vi "Signals.Scale.EU.vi"(4 "Buffer?":bool, 5 "Lookup":variant, 6 "Type":T1, 7 "Reads Ref":T2, 8 "error in (no error)":errorcluster, 10 "Unscaled Data":u8[](array[numeric]), 11 "ID":u32) -> (0 "error out":errorcluster)   [LabVIEW 2019, in "Diagnostics Addon Engine.lvlib"]
uses:
  Diagnostics Addon Engine.lvlib
  <vilib>/NI/NIVS Inline Async API/_Data Access Engine/Data Access Engine/Types/Write.DVR.ctl
  <vilib>/NI/NIVS Inline Async API/_Data Access Engine/Access Type Classes/Write/Write.lvclass
  Shared/Types/Type.ctl
  <vilib>/xnet/xnet.llb/XNET Frame CAN.ctl
  <vilib>/xnet/xnet.llb/XNET Frame Type CAN.ctl
  Shared/Types/Frame.Lookup.Info.ctl
  <vilib>/NI/NIVS Inline Async API/_Data Access Engine/Access Type Classes/Write/Write.lvclass/Write.ctl
  <vilib>/NI/NIVS Inline Async API/_Data Access Engine/Data Access Engine/Methods/Write.Data.Buffer.vi
  <vilib>/NI/NIVS Inline Async API/_Data Access Engine/Data Access Engine/Methods/Write.Data.vi
  <vilib>/NI/NIVS Inline Async API/_Data Access Engine/Access Type Classes/Write/Write.Buffer.vi
  <vilib>/NI/NIVS Inline Async API/_Data Access Engine/Access Type Classes/Write/Write.ProcessData.vi
  Shared/SubVIs/Constants.vi
  <vilib>/xnet/xnet.llb/XNET Convert (Frame CAN to Signal).vi
  Shared/Diagnostics Addon Shared.lvlib
  <vilib>/NI VeriStand/Custom Device Tools/Custom Device Utility Library/Custom Device Utility Library.lvlib
  <vilib>/NI/NIVS Inline Async API/_Data Access Engine/Data Access Engine/Data Access Engine.lvclass
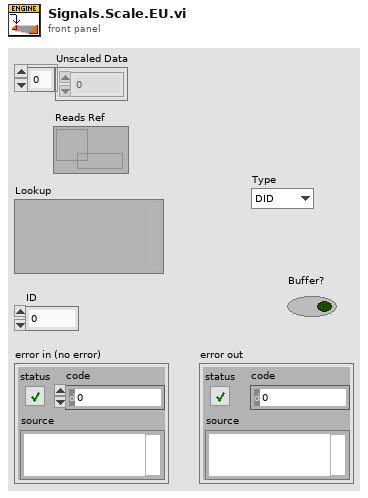
[diagram p1: front panel]
types:
  T1 = typedef "Diagnostics Addon Shared.lvlib/Type.ctl" = enum16{"DID", "CDID", "PID", "CPID", "Read Memory", "Write Memory", "IO Control", "Routine Start", "Routine Request", "Routine Stop", "User Defined", "DTC Control", "Clear DTCs", "Read DTCs", "Start DTCs", "DTC Change Count", "Tester Present", "Unlock ECU", "Reset ECU", "Diag Session Control", "Communication Control", "DPID Control", "Poll Control", "Diag CAN Control"}
  T2 = typedef "Data Access Engine.lvlib/Data Access Engine.lvclass/Write.DVR.ctl" = refnum<data-value>
  T3 = enum16{"Output/Write", "Input/Read", "Input/ReadWrite"}
  T4 = typedef "XNET Frame CAN.ctl" = cluster{"timestamp":timestamp, "payload":u8[], "identifier":u32, "type":T5, "extended?":bool, "echo?":bool}
  T5 = typedef "XNET Frame Type CAN.ctl" = u8
  T6 = typedef "Diagnostics Addon Shared.lvlib/Frame.Lookup.Info.ctl" = cluster{"Offset":i32, "Length":i32, "ByteLength":u16}
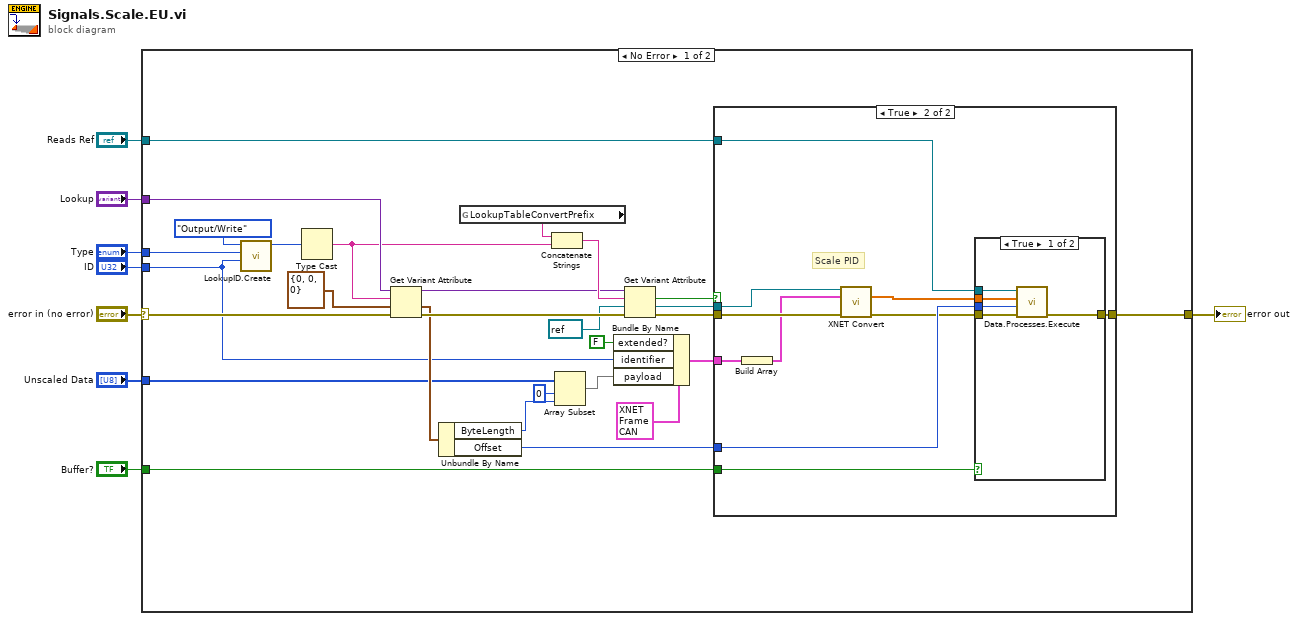
[diagram p0: block diagram]
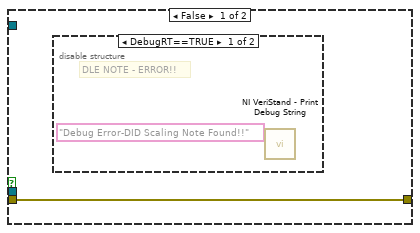
[diagram p2: hidden frame]
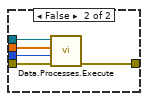
[diagram p4: hidden frame]
diagram:
  n1 = case shown="No Error" "error in (no error)" {
    selector: "error in (no error)" -> [w33 w58]
    tunnel: "Reads Ref" -> [w35 _]
    tunnel: "Lookup" -> [w32 _]
    tunnel: [w34 w58] -> w6
    tunnel: "Unscaled Data" -> [w14 _]
    tunnel: "ID" -> [w11 _]
    tunnel: "Type" -> [w12 _]
    tunnel: "Buffer?" -> [w17 _]
    frame No Error {
      n2 = call "LookupID.Create.vi"("Serivce ID"=w11, "Service Type"=w12, "Direction"=T3."Output/Write") -> ("Result"=w9:u64)  [unwired: 8 in]
      n3 = Type Cast(x=w9) -> (*(type *) &x=w23:string)  [unwired: 1 in]
      n4 = Get Variant Attribute(Variant=w32, name=w23, default value (empty Variant)=T6 {"Offset"=0, "Length"=0, "ByteLength"=0} ("cluster"), error in=w33) -> (duplicate Variant=w21:variant, value=w25:T6)  [unwired: 2 out]
      n5 = Unbundle By Name(w25) -> ("ByteLength"=w16:u16, "Offset"=w15:i32)
      n6 = global read "Constants.vi" "LookupTableConvertPrefix"() -> (w31:string)
      n7 = Concatenate Strings(w31, w23) -> (w29:string)
      n8 = Array Subset(array=w14, index=0, length=w16) -> (w13:u8[])
      n9 = Bundle By Name(cluster=T4 {"timestamp"=timestamp(0 s since 1904-01-01), "payload"=[], "identifier"=0, "type"=0, "extended?"=FALSE, "echo?"=FALSE} ("CAN frame"), "extended?"=FALSE, "identifier"=w11, "payload"=w13) -> (w19:T4)
      n10 = Get Variant Attribute(Variant=w21, name=w29, default value (empty Variant)=refnum<k21> refnum ("DID Conversion"), error in=w33) -> (found=w26:bool, value=w27:refnum<k21>, error out=w30:errorcluster)  [unwired: 1 out]
      n11 = case shown="True" w26 {
        tunnel: w35 -> [_ w41]
        tunnel: [w36 w39] -> w34
        tunnel: w30 -> [w36 w47]
        tunnel: w27 -> [_ w46]
        tunnel: w15 -> [_ w43]
        tunnel: w19 -> [_ w45]
        tunnel: w17 -> [_ w38]
        frame False {
          n12 = disable-structure shown="DebugRT==TRUE" {
            frame condition #0 {
              # "DLE NOTE - ERROR!!"
              n13 = call <vilib>:"NI VeriStand - Print Debug String.vi"("Message"="Debug Error-DID Scaling Note Found!!" ("Debug String")) -> ()  [unwired: 10 in, 1 out]
            }
            frame condition #1 (active) {
            }
          }
        }
        frame True {
          # "Scale PID"
          n14 = Build Array(w45) -> (w44:T4[])
          n15 = call-poly <vilib>:"XNET Convert.vi"("session in"=w46, "frame data"=w44, "error in (no error)"=w47) -> ("signal data"=w42:dbl[], "error out"=w40:errorcluster)  [unwired: 10 in, 1 out]
          n16 = case shown="True" w38 {
            tunnel: w43 -> [w52 w57]
            tunnel: w42 -> [w51 w56]
            tunnel: w41 -> [w50 w53]
            tunnel: w40 -> [w49 w55]
            tunnel: [w48 w54] -> w39
            frame True {
              n17 = call-poly <vilib>:"Data.Processes.Execute.vi"("error in (no error)"=w49, "Offset"=w52, "Values"=w51, "Ref"=w50) -> ("error out"=w48:errorcluster)  [unwired: 7 in]
            }
            frame False {
              n18 = call-poly <vilib>:"Data.Processes.Execute.vi"("error in (no error)"=w55, "Offset"=w57, "Values"=w56, "Ref"=w53) -> ("error out"=w54:errorcluster)  [unwired: 7 in]
            }
          }
        }
      }
    }
    frame Error {
    }
  }
  "error out" <- w6
